vi "Stepper Close.vi"(7 "Stepper #":u8, 8 "error in":errorcluster, 11 "Arduino Resource":T1={"VISA resource"="", "Board Type"=enum."Arduino Uno", "Connection Type"=enum."USB / Serial", "Bytes Per Packet (15)"=15}) -> (0 "error out":errorcluster, 3 "Arduino Resource Out":T1={"VISA resource"="", "Board Type"=enum."Arduino Uno", "Connection Type"=enum."USB / Serial", "Bytes Per Packet (15)"=15})   [LabVIEW 2011, in "LabVIEW Interface for Arduino.lvlib"]
doc: "Sets stepper control pins to low. Depending on the stepper driver this may or may not reduce motor power consumption."
uses:
  LabVIEW Interface for Arduino.lvlib
  Private/Type Defs/Arduino Resource.ctl
  Private/Type Defs/Board Type.ctl
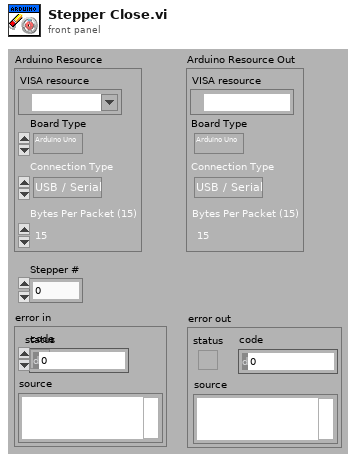
[diagram p1: front panel]
types:
  T1 = typedef "LabVIEW Interface for Arduino.lvlib/Arduino Resource.ctl" = cluster{"VISA resource":refnum<visa-resource-name>, "Board Type":T2, "Connection Type":enum8{"USB / Serial"}, "Bytes Per Packet (15)":u8}
  T2 = typedef "LabVIEW Interface for Arduino.lvlib/Board Type.ctl" = enum16{"Arduino Uno", "Dimuelanove w/Atmega 328", "Mega 2560", "Chipkit Uno32", "Chipkit Max32"}
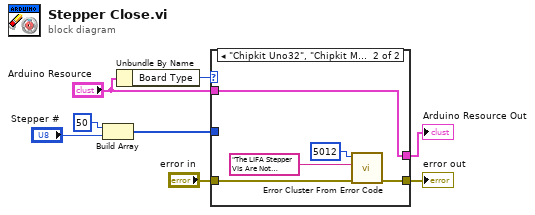
[diagram p0: block diagram]
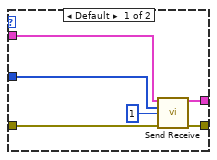
[diagram p2: hidden frame]
diagram:
  n1 = Build Array(u8 50, "Stepper #") -> (w2:u8[])
  n2 = Unbundle By Name("Arduino Resource") -> ("Board Type"=w6:T2)
  n3 = case shown="\"Chipkit Uno32\", \"Chipkit Max32\"" w6 {
    tunnel: "error in" -> [w13 w17]
    tunnel: [w11 w16] -> w3
    tunnel: "Arduino Resource" -> [w12 w15]
    tunnel: w2 -> [w10 _]
    tunnel: [w9 w15] -> w1
    frame Default {
      n4 = call "Send Receive.vi"("Arduino Resource"=w12, "Data"=w10, "Bytes To Read (0)"=u8 1, "error in"=w13) -> ("Arduino Resource"=w9:T1, "error out"=w11:errorcluster)  [unwired: 9 in, 1 out]
    }
    frame "Chipkit Uno32", "Chipkit Max32" {
      n5 = call <vilib>:"Error Cluster From Error Code.vi"("error in (no error)"=w17, "error message (\"\")"="The LIFA Stepper VIs Are Not Supported On Chipkit Targets." ("source"), "error code (0)"=5012) -> ("error out"=w16:errorcluster)  [unwired: 6 in]
    }
  }
  "Arduino Resource Out" <- w1
  "error out" <- w3
